vi "Spin pumping SR830.vi"() -> ()   [LabVIEW 2019]
panel:
  in  "SR830":T1
  in  "AM Depth (%)":dbl
  in  "AM Freq (Hz)":dbl
  in  "Multicolumn Listbox":i32(listbox)
  in  "# of pt":dbl
  in  "Kepco Max I":dbl
  out "XY Graph":cluster{"X":dbl, "Y":dbl}[](graph)
  in  "Kepco GPIB Addr 2":dbl
  in  "SMB 100a GPIB Addr":dbl
  in  "SR830 GPIB Addr":dbl
  in  "Model 7010 GPIB Addr":dbl
  in  "stop":bool
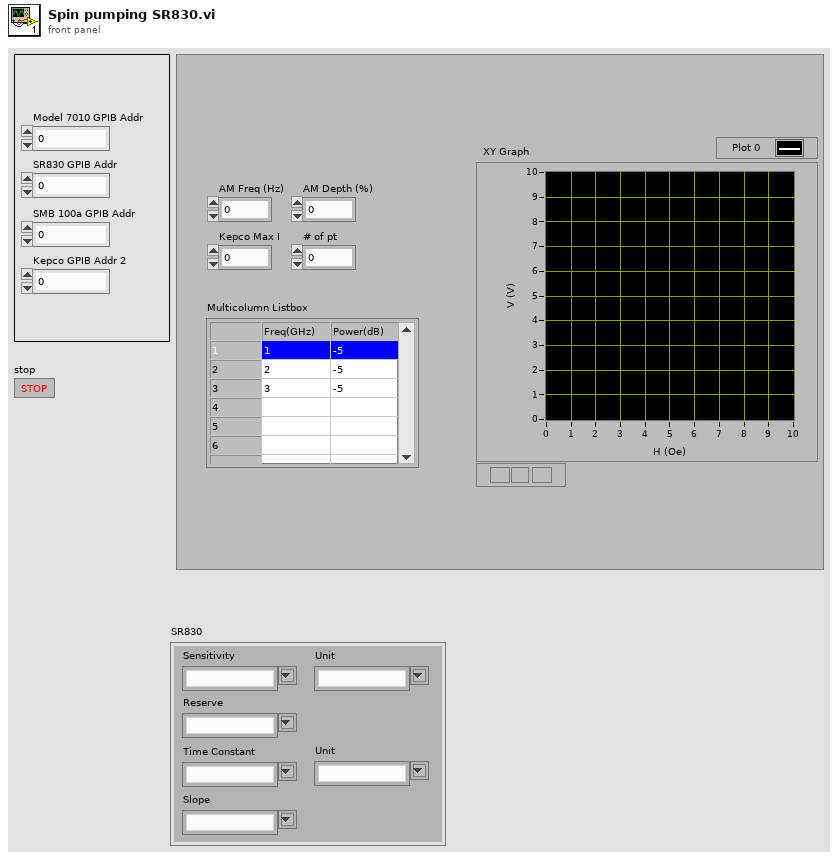
[diagram p1: front panel]
types:
  T1 = cluster{"Sensitivity":string, "Unit":string, "Reserve":string, "Time Constant":string, "Unit":string, "Slope":string}
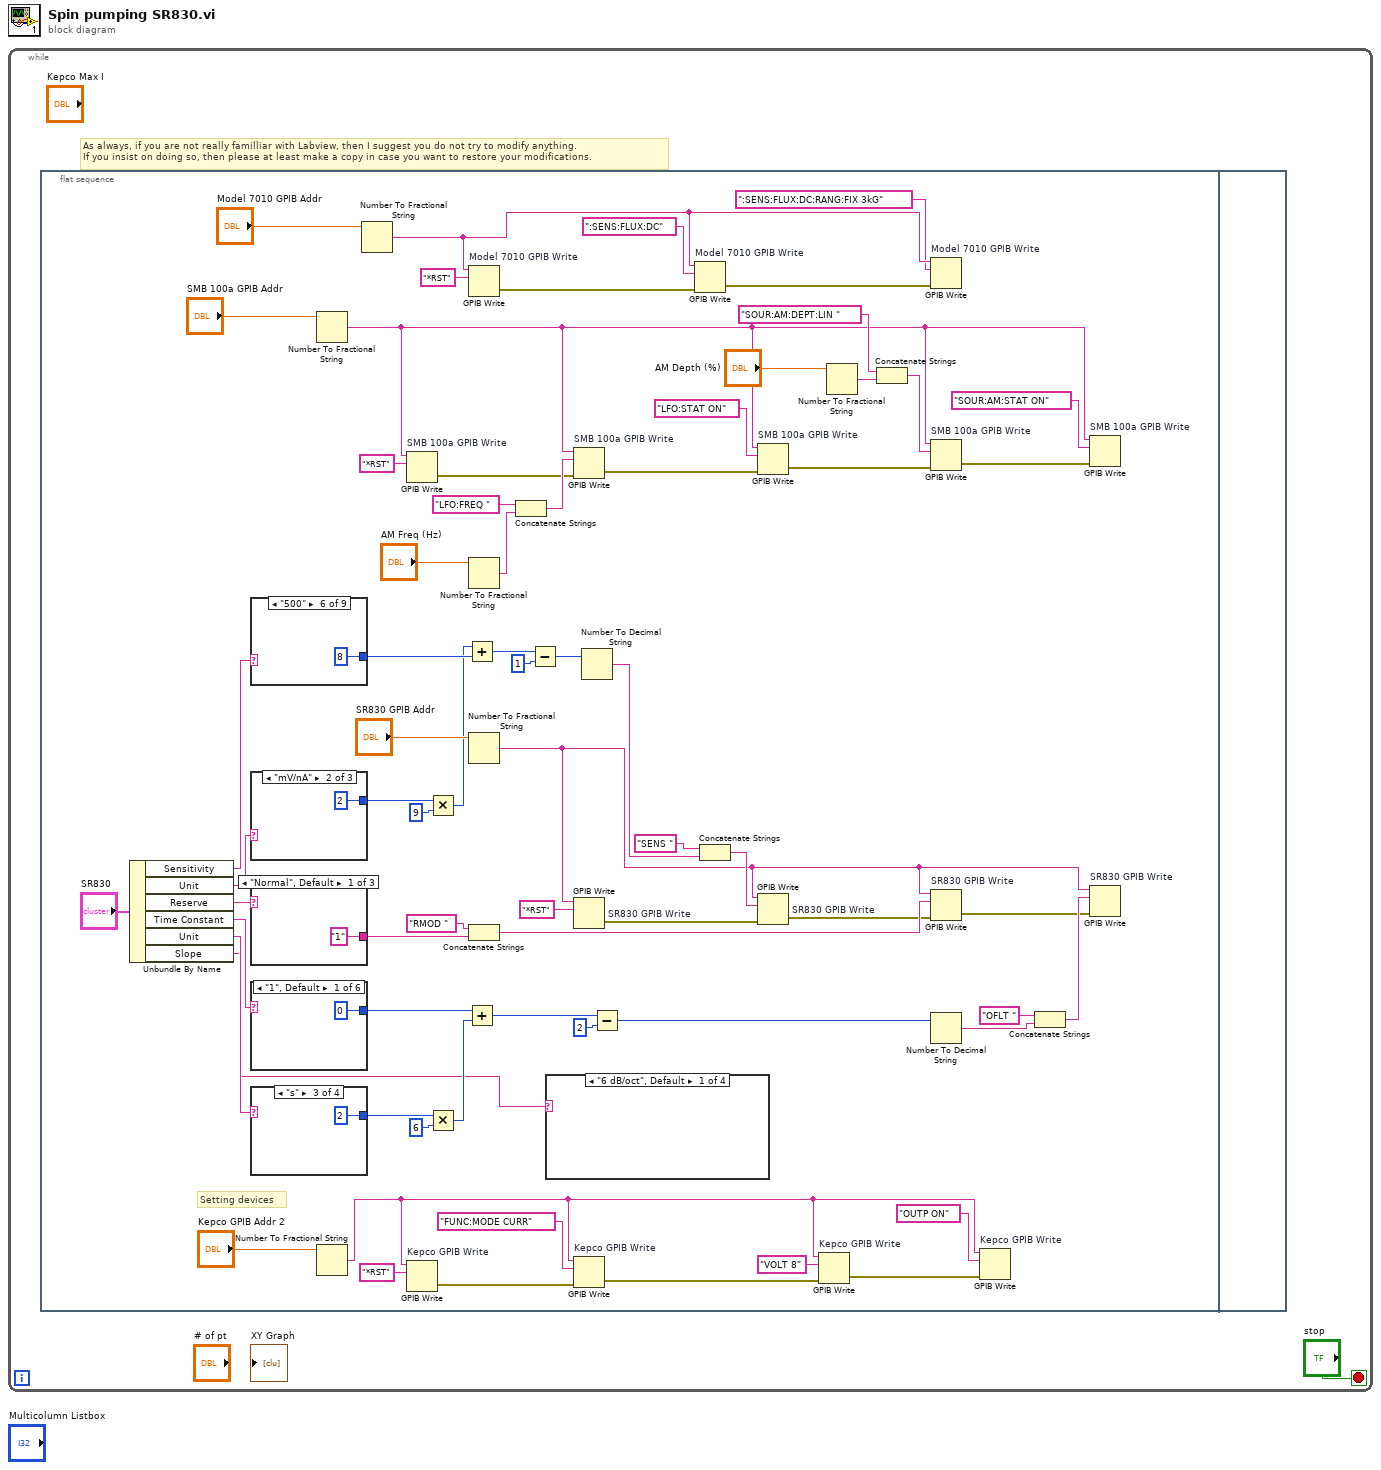
[diagram p0: block diagram]
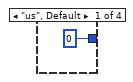
[diagram p5: hidden frame]
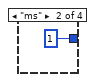
[diagram p6: hidden frame]
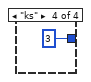
[diagram p7: hidden frame]
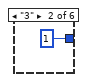
[diagram p8: hidden frame]
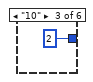
[diagram p9: hidden frame]
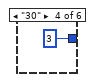
[diagram p10: hidden frame]
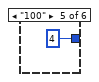
[diagram p11: hidden frame]
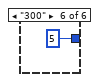
[diagram p12: hidden frame]
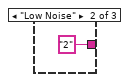
[diagram p13: hidden frame]
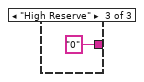
[diagram p14: hidden frame]
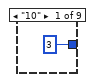
[diagram p15: hidden frame]
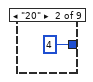
[diagram p16: hidden frame]
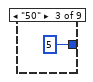
[diagram p17: hidden frame]
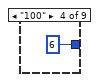
[diagram p18: hidden frame]
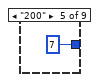
[diagram p19: hidden frame]
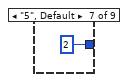
[diagram p20: hidden frame]
diagram:
  n1 = while {
    stop <- "stop" stop-if-true
    # "As always, if you are not really familliar with Labview, then I suggest you do not try to modify anything.\nIf you insist on doing so, then please at least make a copy in case you want to restore your modifications."
    n2 = flat-sequence {
      frame #0 {
        # "Setting devices"
        n3 = Unbundle By Name("SR830") -> ("Sensitivity"=w32:string, "Unit"=w33:string, "Reserve"=w21:string, "Time Constant"=w16:string, "Unit"=w15:string, "Slope"=w2:string)
        n4 = case shown="\"500\"" w32 {
          tunnel: [3 4 5 6 7 8 2 0 1] -> w31
          frame "10" {
          }
          frame "20" {
          }
          frame "50" {
          }
          frame "100" {
          }
          frame "200" {
          }
          frame "500" {
          }
          frame "5", Default {
          }
          frame "1" {
          }
          frame "2" {
          }
        }
        n5 = case shown="\"mV/nA\"" w33 {
          tunnel: [0 2 1] -> w24
          frame "nV/fA", Default {
          }
          frame "mV/nA" {
          }
          frame "uV/pA" {
          }
        }
        n6 = case shown="\"Normal\", Default" w21 {
          tunnel: ["1" "2" "0"] -> w20
          frame "Normal", Default {
          }
          frame "Low Noise" {
          }
          frame "High Reserve" {
          }
        }
        n7 = case shown="\"1\", Default" w16 {
          tunnel: [0 1 2 3 4 5] -> w11
          frame "1", Default {
          }
          frame "3" {
          }
          frame "10" {
          }
          frame "30" {
          }
          frame "100" {
          }
          frame "300" {
          }
        }
        n8 = case shown="\"s\"" w15 {
          tunnel: [0 1 2 3] -> w14
          frame "us", Default {
          }
          frame "ms" {
          }
          frame "s" {
          }
          frame "ks" {
          }
        }
        n9 = Number To Fractional String(number="SMB 100a GPIB Addr") -> (F-format string=w46:string)  [unwired: 3 in]
        n10 = Number To Fractional String(number="Kepco GPIB Addr 2") -> (F-format string=w61:string)  [unwired: 3 in]
        n11 = Number To Fractional String(number="Model 7010 GPIB Addr") -> (F-format string=w41:string)  [unwired: 3 in]
        n12 = GPIB Write "SMB 100a GPIB Write"(0:w46, 1:"*RST" ("data")) -> (6:w55:errorcluster)  [unwired: 3 in, 1 out]
        n13 = GPIB Write "Kepco GPIB Write"(0:w61, 1:"*RST" ("data")) -> (6:w66:errorcluster)  [unwired: 3 in, 1 out]
        n14 = Multiply(x=w24, y=9) -> (x*y=w22:i32)
        n15 = Multiply(x=w14, y=6) -> (x*y=w12:i32)
        n16 = Add(x=w22, y=w31) -> (x+y=w30:i32)
        n17 = Add(x=w11, y=w12) -> (x+y=w9:i32)
        n18 = GPIB Write "Model 7010 GPIB Write"(0:w41, 1:"*RST" ("data")) -> (6:w44:errorcluster)  [unwired: 3 in, 1 out]
        n19 = Number To Fractional String(number="AM Freq (Hz)") -> (F-format string=w58:string)  [unwired: 3 in]
        n20 = Number To Fractional String(number="SR830 GPIB Addr") -> (F-format string=w4:string)  [unwired: 3 in]
        n21 = Concatenate Strings("RMOD " ("string"), w20) -> (w18:string)
        n22 = Concatenate Strings("LFO:FREQ " ("string"), w58) -> (w56:string)
        n23 = Subtract(x=w30, y=1) -> (x-y=w28:i32)
        n24 = case shown="\"6 dB/oct\", Default" w2 {
          frame "6 dB/oct", Default {
          }
          frame "12 dB/oct" {
          }
          frame "18 dB/oct" {
          }
          frame "24 dB/oct" {
          }
        }
        n25 = GPIB Write "SMB 100a GPIB Write"(0:w46, 1:w56, 3:w55) -> (6:w54:errorcluster)  [unwired: 2 in, 1 out]
        n26 = GPIB Write "SR830 GPIB Write"(0:w4, 1:"*RST" ("data")) -> (6:w35:errorcluster)  [unwired: 3 in, 1 out]
        n27 = GPIB Write "Kepco GPIB Write"(0:w61, 1:"FUNC:MODE CURR" ("data"), 3:w66) -> (6:w64:errorcluster)  [unwired: 2 in, 1 out]
        n28 = Number To Decimal String(number=w28) -> (decimal integer string=w27:string)  [unwired: 1 in]
        n29 = Subtract(x=w9, y=2) -> (x-y=w8:i32)
        n30 = GPIB Write "Model 7010 GPIB Write"(0:w41, 1:":SENS:FLUX:DC" ("data"), 3:w44) -> (6:w42:errorcluster)  [unwired: 2 in, 1 out]
        n31 = Concatenate Strings("SENS " ("string"), w27) -> (w25:string)
        n32 = GPIB Write "SMB 100a GPIB Write"(0:w46, 1:"LFO:STAT ON" ("data"), 3:w54) -> (6:w51:errorcluster)  [unwired: 2 in, 1 out]
        n33 = GPIB Write "SR830 GPIB Write"(0:w4, 1:w25, 3:w35) -> (6:w17:errorcluster)  [unwired: 2 in, 1 out]
        n34 = GPIB Write "Kepco GPIB Write"(0:w61, 1:"VOLT 8" ("data"), 3:w64) -> (6:w62:errorcluster)  [unwired: 2 in, 1 out]
        n35 = Number To Fractional String(number="AM Depth (%)") -> (F-format string=w50:string)  [unwired: 3 in]
        n36 = Concatenate Strings("SOUR:AM:DEPT:LIN " ("string"), w50) -> (w49:string)
        n37 = GPIB Write "Model 7010 GPIB Write"(0:w41, 1:":SENS:FLUX:DC:RANG:FIX 3kG" ("data"), 3:w42) -> ()  [unwired: 2 in, 2 out]
        n38 = GPIB Write "SMB 100a GPIB Write"(0:w46, 1:w49, 3:w51) -> (6:w47:errorcluster)  [unwired: 2 in, 1 out]
        n39 = GPIB Write "SR830 GPIB Write"(0:w4, 1:w18, 3:w17) -> (6:w3:errorcluster)  [unwired: 2 in, 1 out]
        n40 = Number To Decimal String(number=w8) -> (decimal integer string=w7:string)  [unwired: 1 in]
        n41 = GPIB Write "Kepco GPIB Write"(0:w61, 1:"OUTP ON" ("data"), 3:w62) -> ()  [unwired: 2 in, 2 out]
        n42 = Concatenate Strings("OFLT " ("string"), w7) -> (w5:string)
        n43 = GPIB Write "SMB 100a GPIB Write"(0:w46, 1:"SOUR:AM:STAT ON" ("data"), 3:w47) -> ()  [unwired: 2 in, 2 out]
        n44 = GPIB Write "SR830 GPIB Write"(0:w4, 1:w5, 3:w3) -> ()  [unwired: 2 in, 2 out]
      }
      frame #1 {
      }
    }
  }
